vi "DB_LeePolar_Graficas.vi"(8 "error in (no error)":errorcluster, 11 "ID_EQUIPO":i32=1) -> (0 "error out":errorcluster, 3 "Polar_VI":T1)   [LabVIEW 2018]
uses:
  Controls/Polar_cluster.ctl
  <vilib>/addons/database/Connection.llb/DB Tools Open Connec (Path).vi
  <vilib>/addons/database/Connection.llb/Conn Execute.vi
  <vilib>/addons/database/Recordset.llb/Rec Fetch Recordset Data (R).vi
  <vilib>/addons/database/Recordset.llb/Rec Destroy - Connection.vi
  <vilib>/addons/database/_DB Variant To Data/Database Variant To Data.xnode
  <vilib>/addons/database/NI_Database_API.lvlib
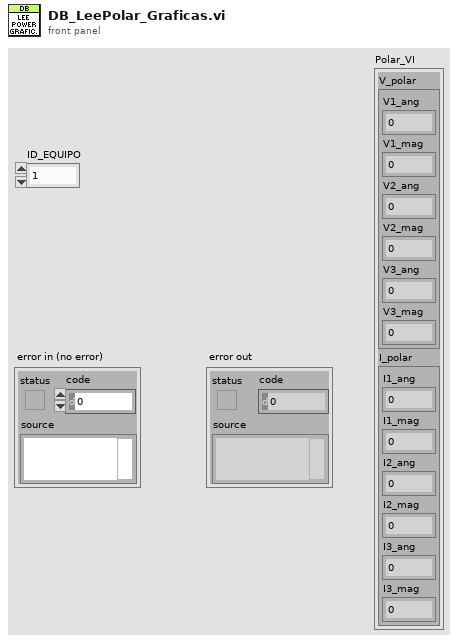
[diagram p1: front panel]
types:
  T1 = typedef "Polar_cluster.ctl" = cluster{"V_polar":cluster{"V1_ang":sgl, "V1_mag":sgl, "V2_ang":sgl, "V2_mag":sgl, "V3_ang":sgl, "V3_mag":sgl}, "I_polar":cluster{"I1_ang":sgl, "I1_mag":sgl, "I2_ang":sgl, "I2_mag":sgl, "I3_ang":sgl, "I3_mag":sgl}}
  T2 = cluster{"I1_ang":sgl, "I1_mag":sgl, "I2_ang":sgl, "I2_mag":sgl, "I3_ang":sgl, "I3_mag":sgl}
  T3 = cluster{"V1_ang":sgl, "V1_mag":sgl, "V2_ang":sgl, "V2_mag":sgl, "V3_ang":sgl, "V3_mag":sgl}
  T4 = typedef "NI_Database_API.lvlib/Conn ObjectReference.ctl" = refnum<k1>
  T5 = typedef "NI_Database_API.lvlib/Rec ObjectReference.ctl" = refnum<k1>
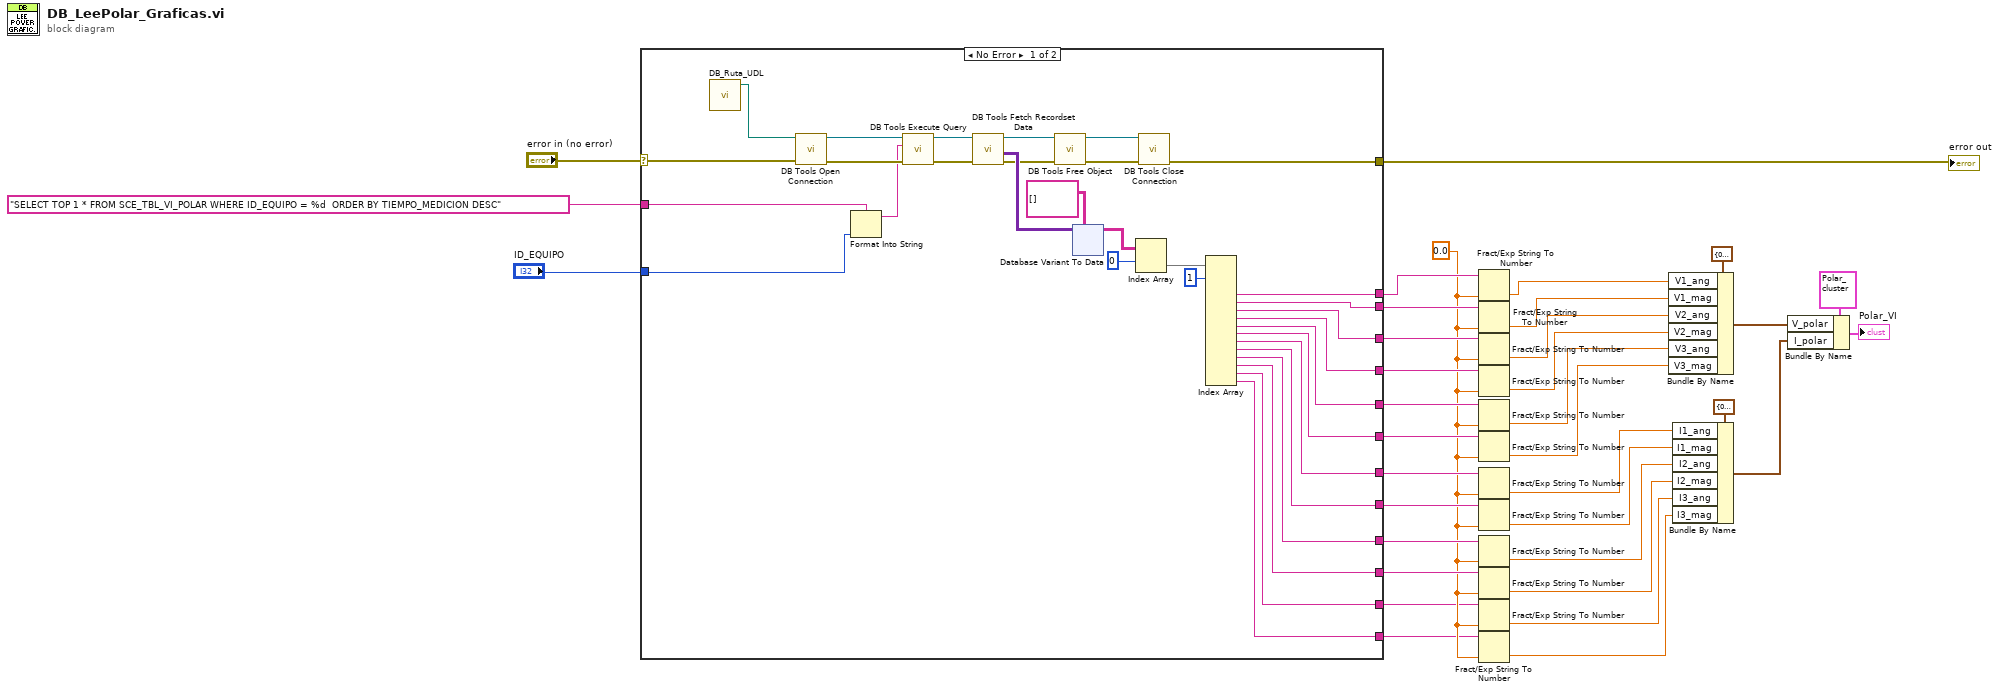
[diagram p0: block diagram]
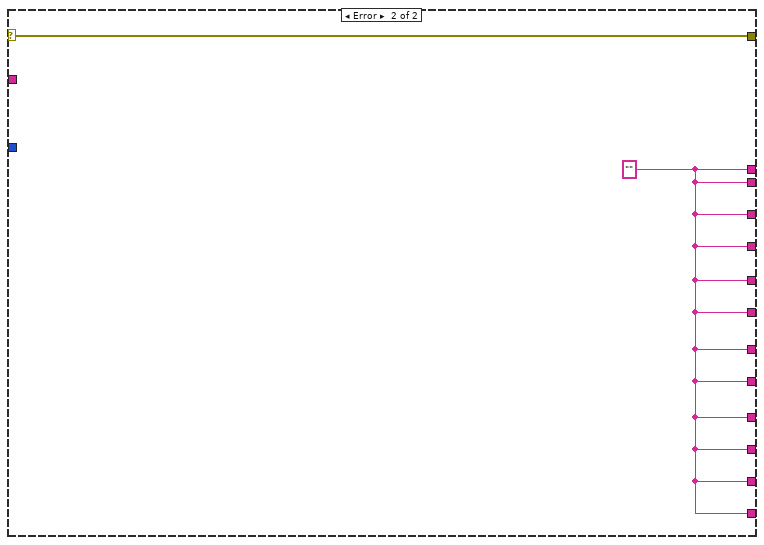
[diagram p2: hidden frame]
diagram:
  w3 = sgl 0.0
  n1 = case shown="No Error" "error in (no error)" {
    selector: "error in (no error)" -> [w62 w113]
    tunnel: [w64 w113] -> w33
    tunnel: "SELECT TOP 1 * FROM SCE_TBL_VI_POLAR WHERE ID_EQUIPO = %d  ORDER BY TIEMPO_MEDICION DESC" ("SQL") -> [w54 _]
    tunnel: [w51 w112] -> w31
    tunnel: [w50 w112] -> w30
    tunnel: [w49 w112] -> w29
    tunnel: "ID_EQUIPO" -> [w52 _]
    tunnel: [w47 w112] -> w28
    tunnel: [w48 w112] -> w27
    tunnel: [w46 w112] -> w26
    tunnel: [w44 w112] -> w21
    tunnel: [w42 w112] -> w10
    tunnel: [w41 w112] -> w8
    tunnel: [w40 w112] -> w7
    tunnel: [w39 w112] -> w2
    tunnel: [w38 w112] -> w1
    frame No Error {
      n2 = call "DB_Ruta_UDL.vi"() -> ("UDL ruta"=w37:path)  [unwired: 11 in]
      n3 = call-poly <vilib>:"DB Tools Open Connection.vi"("error in (no error)"=w62, "connection information"=w37) -> ("error out"=w67:errorcluster, "connection reference"=w65:T4)  [unwired: 6 in]
      n4 = Format Into String(format string=w54, w52) -> (resulting string=w53:string)  [unwired: 2 in, 1 out]
      n5 = call-poly <vilib>:"DB Tools Execute Query.vi"("error in (no error)"=w67, "SQL query"=w53, "connection reference"=w65) -> ("error out"=w63:errorcluster, "recordset reference"=w61:T5)  [unwired: 5 in]
      n6 = call-poly <vilib>:"DB Tools Fetch Recordset Data.vi"("error in (no error)"=w63, "recordset reference"=w61) -> ("error out"=w57:errorcluster, "recordset data"=w58:variant[][], "recordset reference out"=w60:T5)  [unwired: 3 in]
      n7 = call-poly <vilib>:"DB Tools Free Object.vi"("error in (no error)"=w57, "recordset reference"=w60) -> ("error out"=w66:errorcluster, "connection reference"=w36:T4)  [unwired: 8 in]
      n8 = xnode "Database Variant To Data"("database variant"=w58, "type"=string[][] []) -> ("data"=w56:string[][])  [unwired: 1 in, 1 out]
      n9 = Index Array(array=w56, index (row)=0 ("disabled index (col)")) -> (element=w43:string[])  [unwired: 1 in]
      n10 = call <vilib>:"DB Tools Close Connection.vi"("error in (no error)"=w66, "connection reference"=w36) -> ("error out"=w64:errorcluster)  [unwired: 5 in]
      n11 = Index Array(array=w43, index #1=1 ("index")) -> (element #3=w51:string, element #4=w50:string, element #5=w49:string, element #6=w44:string, element #7=w47:string, element #8=w48:string, element #9=w46:string, element #10=w42:string, element #11=w41:string, element #12=w40:string, element #13=w39:string, element #14=w38:string)  [unwired: 13 in, 2 out]
    }
    frame Error {
      w112 = ""
    }
  }
  "error out" <- w33
  n12 = Fract/Exp String To Number(string=w31, default (0 dbl)=w3) -> (number=w24:sgl)  [unwired: 2 in, 1 out]
  n13 = Fract/Exp String To Number(string=w30, default (0 dbl)=w3) -> (number=w23:sgl)  [unwired: 2 in, 1 out]
  n14 = Fract/Exp String To Number(string=w29, default (0 dbl)=w3) -> (number=w22:sgl)  [unwired: 2 in, 1 out]
  n15 = Fract/Exp String To Number(string=w21, default (0 dbl)=w3) -> (number=w20:sgl)  [unwired: 2 in, 1 out]
  n16 = Fract/Exp String To Number(string=w28, default (0 dbl)=w3) -> (number=w14:sgl)  [unwired: 2 in, 1 out]
  n17 = Fract/Exp String To Number(string=w27, default (0 dbl)=w3) -> (number=w13:sgl)  [unwired: 2 in, 1 out]
  n18 = Fract/Exp String To Number(string=w26, default (0 dbl)=w3) -> (number=w12:sgl)  [unwired: 2 in, 1 out]
  n19 = Fract/Exp String To Number(string=w10, default (0 dbl)=w3) -> (number=w11:sgl)  [unwired: 2 in, 1 out]
  n20 = Fract/Exp String To Number(string=w8, default (0 dbl)=w3) -> (number=w9:sgl)  [unwired: 2 in, 1 out]
  n21 = Fract/Exp String To Number(string=w7, default (0 dbl)=w3) -> (number=w6:sgl)  [unwired: 2 in, 1 out]
  n22 = Fract/Exp String To Number(string=w2, default (0 dbl)=w3) -> (number=w5:sgl)  [unwired: 2 in, 1 out]
  n23 = Fract/Exp String To Number(string=w1, default (0 dbl)=w3) -> (number=w4:sgl)  [unwired: 2 in, 1 out]
  n24 = Bundle By Name(cluster=T3 {"V1_ang"=0.0, "V1_mag"=0.0, "V2_ang"=0.0, "V2_mag"=0.0, "V3_ang"=0.0, "V3_mag"=0.0} ("V_polar"), "V1_ang"=w24, "V1_mag"=w23, "V2_ang"=w22, "V2_mag"=w20, "V3_ang"=w14, "V3_mag"=w13) -> (w25:T3)
  n25 = Bundle By Name(cluster=T2 {"I1_ang"=0.0, "I1_mag"=0.0, "I2_ang"=0.0, "I2_mag"=0.0, "I3_ang"=0.0, "I3_mag"=0.0} ("I_polar"), "I1_ang"=w12, "I1_mag"=w11, "I2_ang"=w9, "I2_mag"=w6, "I3_ang"=w5, "I3_mag"=w4) -> (w16:T2)
  n26 = Bundle By Name(cluster=T1 {"V_polar"={"V1_ang"=0.0, "V1_mag"=0.0, "V2_ang"=0.0, "V2_mag"=0.0, "V3_ang"=0.0, "V3_mag"=0.0}, "I_polar"={"I1_ang"=0.0, "I1_mag"=0.0, "I2_ang"=0.0, "I2_mag"=0.0, "I3_ang"=0.0, "I3_mag"=0.0}} ("Polar_cluster"), "V_polar"=w25, "I_polar"=w16) -> (→"Polar_VI":T1)
